vi "Playback.vi"() -> ()   [LabVIEW 2017]
doc: "This VI reads records of data from the logging table in the LabVIEW.mdb database. \n\nAll the records from the table are retrieved at one time using the DB Tools Select Data VI. This data is in the format of a two dimensional array of variants. This array is indexed and each of the values are converted back to their original data types."
uses:
  database example subvis/Fetching - State.ctl
  <vilib>/addons/database/Connection.llb/Conn ObjectReference.ctl
  <vilib>/addons/database/Connection.llb/DB Tools Open Connec (Path).vi
  <vilib>/addons/database/_DB Variant To Data/Database Variant To Data.xnode
  <vilib>/addons/database/NI_Database_API.lvlib
panel:
  out "data":u8[](array[numeric])
  out "size(s)":i32
  out "record number":i32
  in  "Previous Record":bool
  in  "Next Record":bool
  in  "Stop":bool
  out "min temperature value":dbl format="%#.6g"
  out "max temperature value":dbl format="%#.6g"
  out "min pressure value":dbl format="%#.6g"
  out "max pressure value":dbl format="%#.6g"
  out "Core Temperature":dbl[](graph)
  out "Core Pressure":dbl[](graph)
  # "Overview: Demonstrates how to fetch the contents of an entire table from a database for playback.\nRequirements: Database Connectivity Toolkit\nInstructions:\n1. Make sure you have already run one of the \"Database Logging\" examples.\n2. Run this VI.\n3. Click the Previous Record and Next Record buttons to display individual records from the database.\n4. Click Stop to stop the VI."
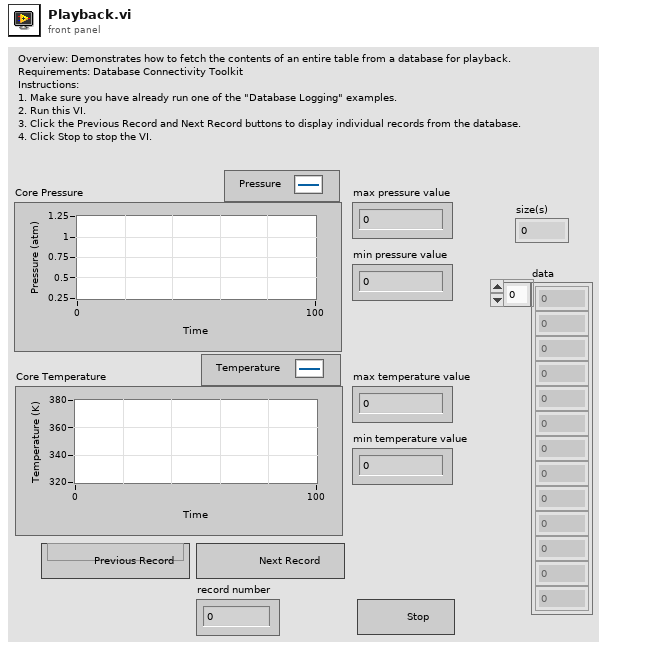
[diagram p1: front panel]
types:
  T1 = typedef "NI_Database_API.lvlib/Conn ObjectReference.ctl" = refnum<k1>
  T2 = typedef "Fetching - State.ctl" = enum16{"Initialize", "Wait for Event", "Prepare for Next", "Prepare for Previous", "Query Database", "Exit"}
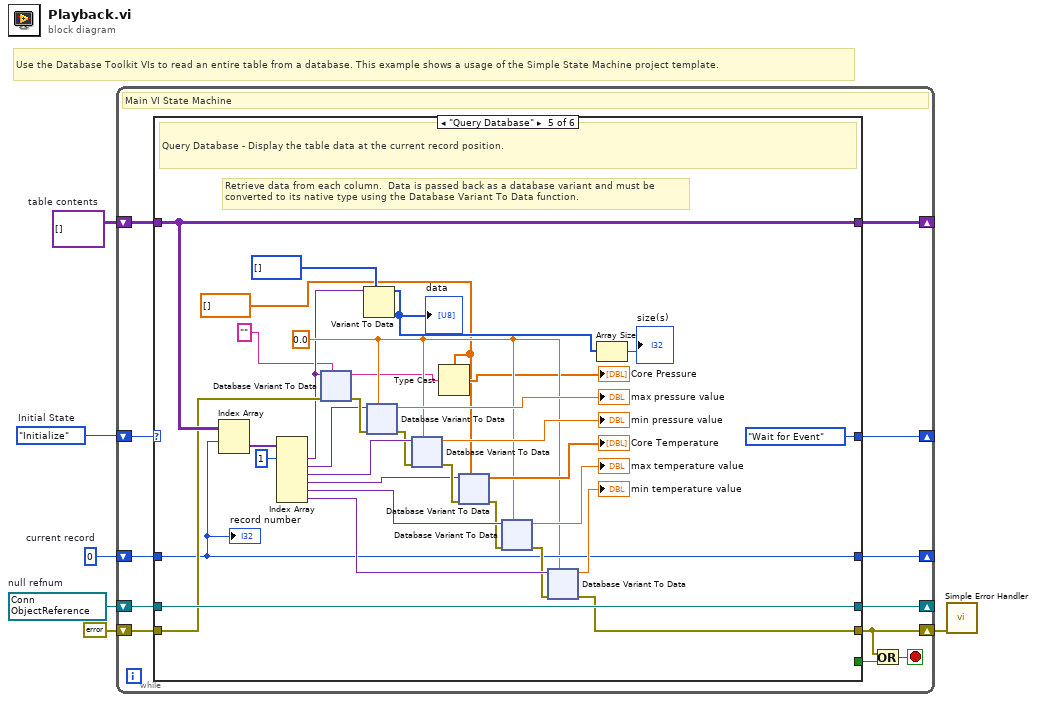
[diagram p0: block diagram]
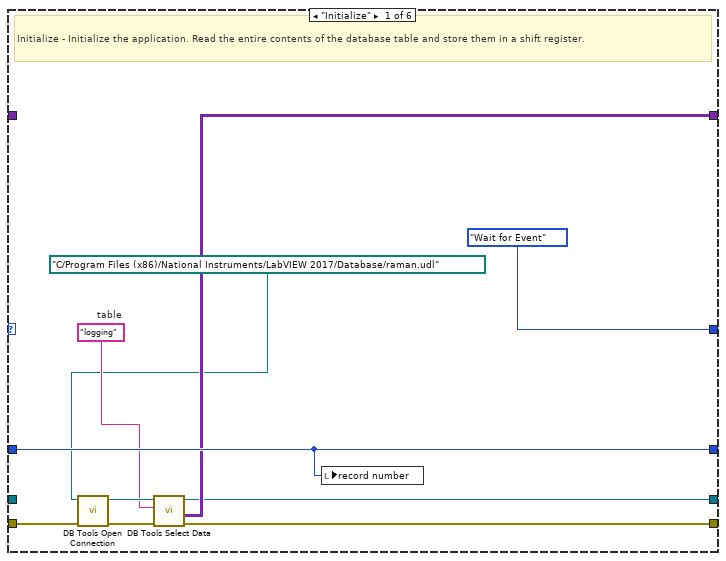
[diagram p2: hidden frame]
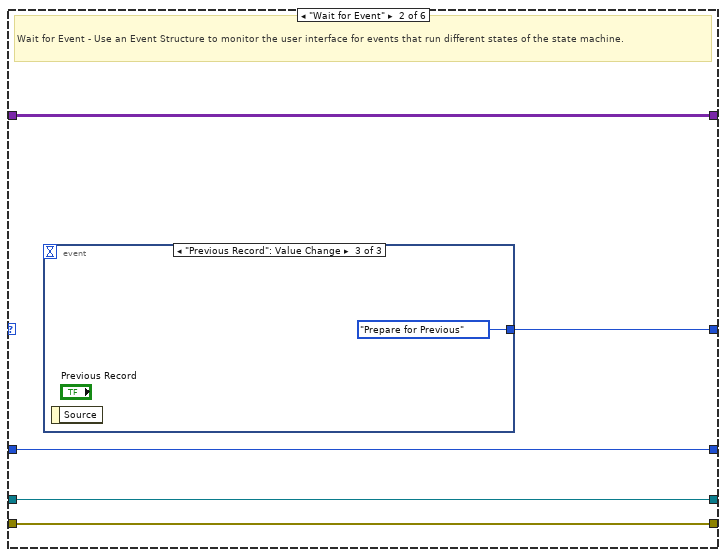
[diagram p3: hidden frame]
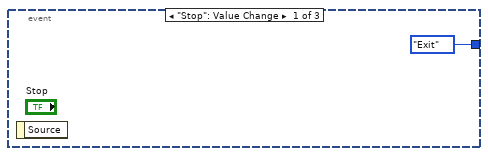
[diagram p4: hidden frame]
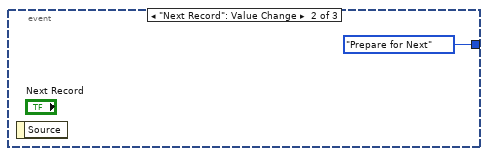
[diagram p5: hidden frame]
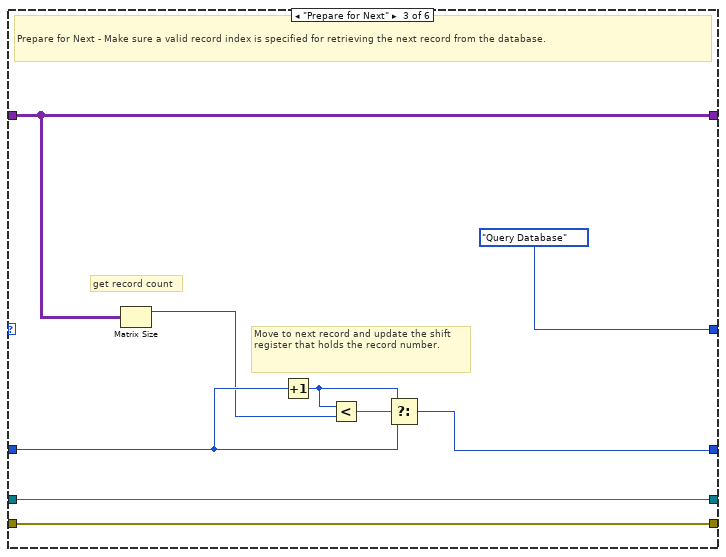
[diagram p6: hidden frame]
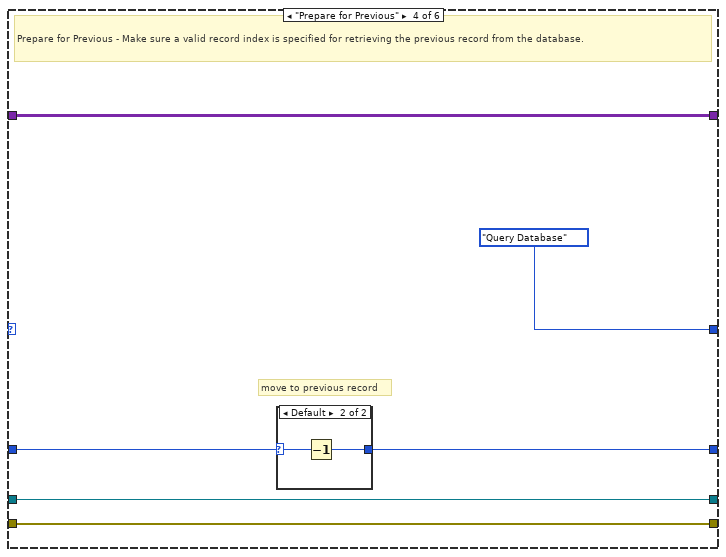
[diagram p7: hidden frame]
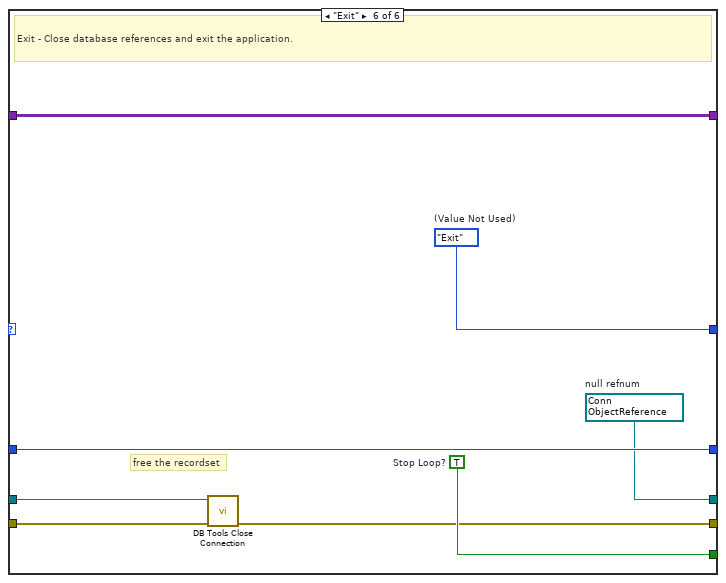
[diagram p9: hidden frame]
diagram:
  w1 = T1 refnum items=["Connection"]  # null refnum
  w2 = variant[][] []  # table contents
  w6 = 0  # current record
  w5 = Fetching_-_State."Initialize"  # Initial State
  # "Use the Database Toolkit VIs to read an entire table from a database. This example shows a usage of the Simple State Machine project template."
  n1 = while {
    shift-right: [w17] -> _
    shift-left: w5 -> [w18]
    shift-right: [w13] -> w3
    shift-left: errorcluster {"status"=FALSE, "code"=0, "source"=""} ("error constant") -> [w16]
    shift-right: [w12] -> _
    shift-left: w1 -> [w11]
    shift-right: [w9] -> _
    shift-left: w6 -> [w10]
    shift-right: [w8] -> _
    shift-left: w2 -> [w7]
    stop <- w14 stop-if-true
    # "Main VI State Machine"
    n2 = case shown="\"Query Database\"" w18 {
      tunnel: [Fetching_-_State."Wait for Event" ("(Value Not Used)") w33 Fetching_-_State."Query Database" ("(Value Not Used)") Fetching_-_State."Query Database" ("(Value Not Used)") Fetching_-_State."Wait for Event" ("(Value Not Used)") w289] -> w17
      tunnel: [_ _ _ _ _ w288] -> w15
      tunnel: w16 -> [w28 w31 w45 w51 w68 w287]
      tunnel: [w24 w31 w45 w51 w67 w286] -> w13
      tunnel: [w20 w32 w43 w49 w85 w283] -> w12
      tunnel: w11 -> [_ w32 w43 w49 w85 w284]
      tunnel: w10 -> [w26 w30 w39 w47 w66 w285]
      tunnel: [w26 w30 w40 w46 w66 w285] -> w9
      tunnel: [w21 w29 w38 w48 w70 w282] -> w8
      tunnel: w7 -> [_ w29 w38 w48 w70 w282]
      frame "Initialize" {
        w22 = "logging"  # table
        # "Initialize - Initialize the application. Read the entire contents of the database table and store them in a shift register."
        n3 = call-poly <vilib>:"DB Tools Open Connection.vi"("error in (no error)"=w28, "connection information"=path "C:/Program Files (x86)/National Instruments/LabVIEW 2017/Database/raman.udl") -> ("error out"=w25:errorcluster, "connection reference"=w23:T1)  [unwired: 6 in]
        n4 = call <vilib>:"DB Tools Select Data.vi"("error in (no error)"=w25, "table"=w22, "connection reference"=w23) -> ("error out"=w24:errorcluster, "data"=w21:variant[][], "connection reference out"=w20:T1)  [unwired: 3 in]
        n5 = local write "record number"(w26) -> ()
      }
      frame "Wait for Event" {
        # "Wait for Event - Use an Event Structure to monitor the user interface for events that run different states of the state machine."
        n6 = event shown="[2] \"Previous Record\": Value Change" {
          selector: _ -> [_ _ _]
          dyn-events: _ -> [_ _ _]
          timeout: _ -> [_ _ _]
          tunnel: [Fetching_-_State."Exit" ("Next State") Fetching_-_State."Prepare for Next" ("Next State") Fetching_-_State."Prepare for Previous" ("Next State")] -> w33
          event "Stop": Value Change {
            n7 = event-data() -> ()  [unwired: 1 in, 1 out]
          }
          event "Next Record": Value Change {
            n8 = event-data() -> ()  [unwired: 1 in, 1 out]
          }
          event "Previous Record": Value Change {
            n9 = event-data() -> ()  [unwired: 1 in, 1 out]
          }
        }
      }
      frame "Prepare for Next" {
        # "get record count"
        # "Move to next record and update the shift register that holds the record number."
        # "Prepare for Next - Make sure a valid record index is specified for retrieving the next record from the database."
        n10 = Matrix Size(0:w38) -> (1:w37:i32)  [unwired: 1 out]
        n11 = Increment(x=w39) -> (x+1=w42:i32)
        n12 = Less?(x=w42, y=w37) -> (x < y?=w41:bool)
        n13 = Select(t=w42, s=w41, f=w39) -> (s? t:f=w40:i32)
      }
      frame "Prepare for Previous" {
        # "move to previous record"
        # "Prepare for Previous - Make sure a valid record index is specified for retrieving the previous record from the database."
        n14 = case shown="Default" w47 {
          selector: w47 -> [w52 w53]
          tunnel: [w52 w54] -> w46
          frame 0 {
          }
          frame Default {
            n15 = Decrement(x=w53) -> (x-1=w54:i32)
          }
        }
      }
      frame "Query Database" {
        w63 = 0.0
        w55 = dbl[] [] ("Array Constant")
        # "Retrieve data from each column.  Data is passed back as a database variant and must be converted to its native type using the Database Variant To Data function."
        # "Query Database - Display the table data at the current record position."
        n16 = Index Array(array=w70, index (row)=w66) -> (element=w71:variant[])  [unwired: 1 in]
        n17 = Index Array(array=w71, index #1=1) -> (element #1=w61:variant, element #2=w62:variant, element #3=w80:variant, element #4=w81:variant, element #5=w82:variant, element #6=w83:variant)  [unwired: 5 in]
        n18 = xnode "Database Variant To Data"("database variant"=w61, "error in (no error)"=w68, "type"="") -> ("data"=w57:string, "error out"=w79:errorcluster)
        n19 = Variant To Data(type=u8[] [], Variant=w61) -> (data=w60:u8[])  [unwired: 1 in, 1 out]
        "data" <- w60
        n20 = xnode "Database Variant To Data"("database variant"=w62, "error in (no error)"=w79, "type"=w63) -> ("data"=→"max pressure value":dbl, "error out"=w77:errorcluster)
        n21 = xnode "Database Variant To Data"("database variant"=w80, "error in (no error)"=w77, "type"=w63) -> ("data"=→"min pressure value":dbl, "error out"=w84:errorcluster)
        n22 = Type Cast(type=w55, x=w57) -> (*(type *) &x=→"Core Pressure":dbl[])
        n23 = xnode "Database Variant To Data"("database variant"=w81, "error in (no error)"=w84, "type"=w55) -> ("data"=→"Core Temperature":dbl[], "error out"=w78:errorcluster)
        n24 = xnode "Database Variant To Data"("database variant"=w82, "error in (no error)"=w78, "type"=w63) -> ("data"=→"max temperature value":dbl, "error out"=w69:errorcluster)
        n25 = xnode "Database Variant To Data"("database variant"=w83, "error in (no error)"=w69, "type"=w63) -> ("data"=→"min temperature value":dbl, "error out"=w67:errorcluster)
        n26 = Array Size(array=w60) -> (size(s)=→"size(s)":i32)
        "record number" <- w66
      }
      frame "Exit" {
        w283 = T1 refnum items=["Connection"]  # null refnum
        w288 = TRUE  # Stop Loop?
        w289 = Fetching_-_State."Exit"  # (Value Not Used)
        # "free the recordset"
        # "Exit - Close database references and exit the application."
        n27 = call <vilib>:"DB Tools Close Connection.vi"("error in (no error)"=w287, "connection reference"=w284) -> ("error out"=w286:errorcluster)  [unwired: 5 in]
      }
    }
    n28 = Or(x=w13, y=w15) -> (x .or. y?=w14:bool)
  }
  n29 = call <vilib>:"Simple Error Handler.vi"("error in (no error)"=w3) -> ()  [unwired: 4 in, 5 out]
